vi "Read_ADC.vi"(8 "error in (no error)":errorcluster, 10 "CH":i32, 11 "Simulado in":refnum<class "Simulado.lvclass">) -> (0 "error out":errorcluster, 1 "Expected Response":string, 2 "Command to Send":string, 3 "Simulado out":refnum<class "Simulado.lvclass">)   [LabVIEW 2020, in "Simulado.lvclass"]
uses:
  Simulado.lvclass
  Abstract/Serial Device/Combo Box Comandos.ctl
  Abstract/Serial Device/Combo Box Devices.ctl
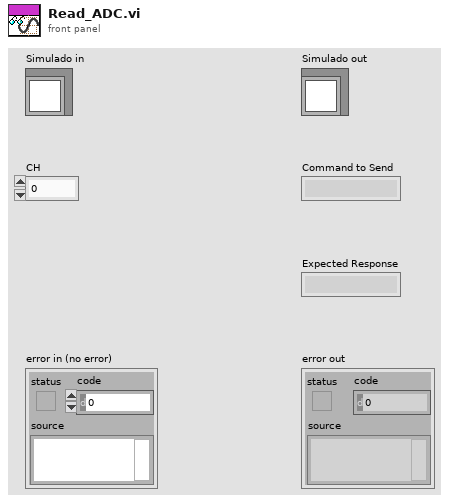
[diagram p1: front panel]
types:
  T1 = typedef "Combo Box Devices.ctl" = string
  T2 = typedef "Combo Box Comandos.ctl" = string
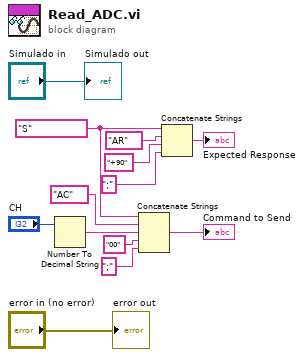
[diagram p0: block diagram]
diagram:
  w10 = T1 "S" ("Serial Devide Brand")
  n1 = Number To Decimal String(number="CH") -> (decimal integer string=w8:string)  [unwired: 1 in]
  n2 = Concatenate Strings(w10, T2 "AC" ("Command"), w8, "00" ("string"), ";" ("string")) -> (→"Command to Send":string)
  n3 = Concatenate Strings(w10, T2 "AR" ("Respuesta"), "+90" ("string"), ";" ("string")) -> (→"Expected Response":string)
  "error out" <- "error in (no error)"
  "Simulado out" <- "Simulado in"
